vi "process.vi"(8 "error in":errorcluster, 9 "result allocation":T2, 10 "parameters":T2, 11 "Simple Sequencer TBM runtime in":refnum<class "Simple Sequencer TBM runtime.lvclass">) -> (0 "error out":errorcluster, 1 "results":T2, 2 "parameter allocation":T2, 3 "Simple Sequencer TBM runtime out":refnum<class "Simple Sequencer TBM runtime.lvclass">)   [LabVIEW 2015, in "Simple Sequencer TBM runtime.lvclass"]
doc: "Provides an interface for information processing by a module at runtime. While this interface performs no operations, a child should provide an override which may process data in any manner necessary."
uses:
  Simple Sequencer TBM runtime.lvclass
  <vilib>/NI/Tag Bus/table/data table.ctl
  sequencer states.ctl
  Simple Sequencer TBM runtime.lvclass/Simple Sequencer TBM runtime.ctl
  sequencer commands.ctl
  meta sequence definition.ctl
  <vilib>/NI/AMC/Read Termination Message.vi
  <vilib>/NI/AMC/Create Single Message.vi
  <vilib>/NI/AMC/Update Message Routing Info.vi
  <vilib>/NI/AMC/Globals.vi
  <vilib>/NI/AMC/Send Message.vi
  <vilib>/NI/AMC/AMC.lvlib
  <vilib>/NI/Tag Bus/table/data table.lvlib
panel:
  out "state":T1
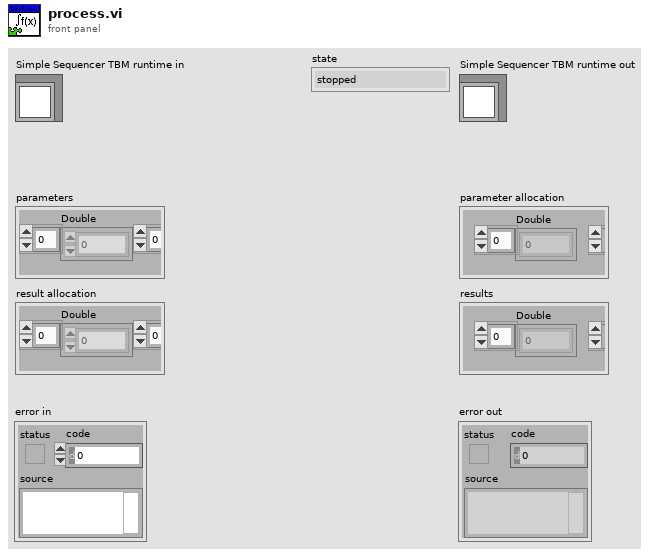
[diagram p1: front panel]
types:
  T1 = typedef "Simple Sequencer TBM runtime.lvclass/sequencer states.ctl" = enum16{"stopped", "running", "paused"}
  T2 = typedef "tag bus.lvlib/data table.lvlib/data table.ctl" = cluster{"Double":dbl[], "Single":sgl[], "I64":i64[], "I32":i32[], "I16":i16[], "I8":i8[], "U64":u64[], "U32":u32[], "U16":u16[], "U8":u8[], "Boolean":bool[], "String":string[], "Array of Double":cluster{"DBL Array":dbl[]}[], "Array of Single":cluster{"SGL Array":sgl[]}[], "Array of I64":cluster{"I64 Array":i64[]}[], "Array of I32":cluster{"I32 Array":i32[]}[], "Array of I16":cluster{"I16 Array":i16[]}[], "Array of I8":cluster{"I8 Array":i8[]}[], "Array of U64":cluster{"U64 Array":u64[]}[], "Array of U32":cluster{"U32 Array":u32[]}[], "Array of U16":cluster{"U16 Array":u16[]}[], "Array of U8":cluster{"U8 Array":u8[]}[], "Array of Boolean":cluster{"Boolean Array":bool[]}[], "Array of String":cluster{"String Array":string[]}[]}
  T3 = typedef "Simple Sequencer TBM runtime.lvclass/sequencer commands.ctl" = enum16{"Run", "Pause", "Resume", "Stop"}
  T4 = typedef "Simple Sequencer TBM runtime.lvclass/meta sequence definition.ctl" = cluster{"sequence length":i32, "sequence pointers":i32[], "continue location":i32}
  T5 = typedef "AMC.lvlib/Message Queue.ctl" = refnum<queue>
  T6 = typedef "Simple Sequencer TBM runtime.lvclass/sequence definition.ctl" = cluster{"sequence name":string, "sequence length":i32, "actions with configuration":T7[]}
  T7 = typedef "Simple Sequencer TBM runtime.lvclass/actions with configuration.ctl" = cluster{"action":refnum<class "action.lvclass">, "parameters":T2, "parameters specification":T8[], "results":T2, "results specification":T8[]}
  T8 = typedef "tag bus.lvlib/data table.lvlib/transfer specification.ctl" = cluster{"data type":T9, "sink indices":i32[], "source indices":i32[]}
  T9 = typedef "tag bus.lvlib/tag descriptor.lvclass/Data Type.ctl" = enum16{"Double", "Single", "I64", "I32", "I16", "I8", "U64", "U32", "U16", "U8", "Boolean", "String", "Array of Double", "Array of Single", "Array of I64", "Array of I32", "Array of I16", "Array of I8", "Array of U64", "Array of U32", "Array of U16", "Array of U8", "Array of Boolean", "Array of String"}
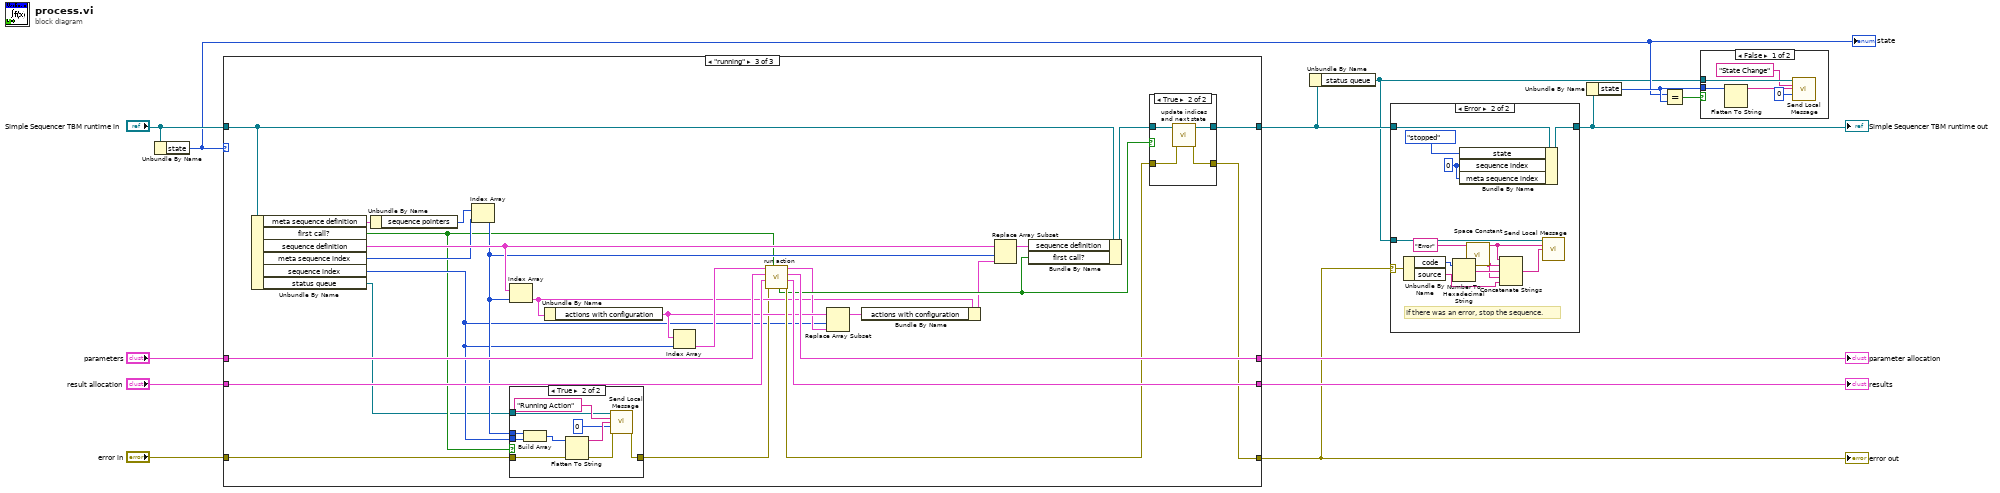
[diagram p0: block diagram]
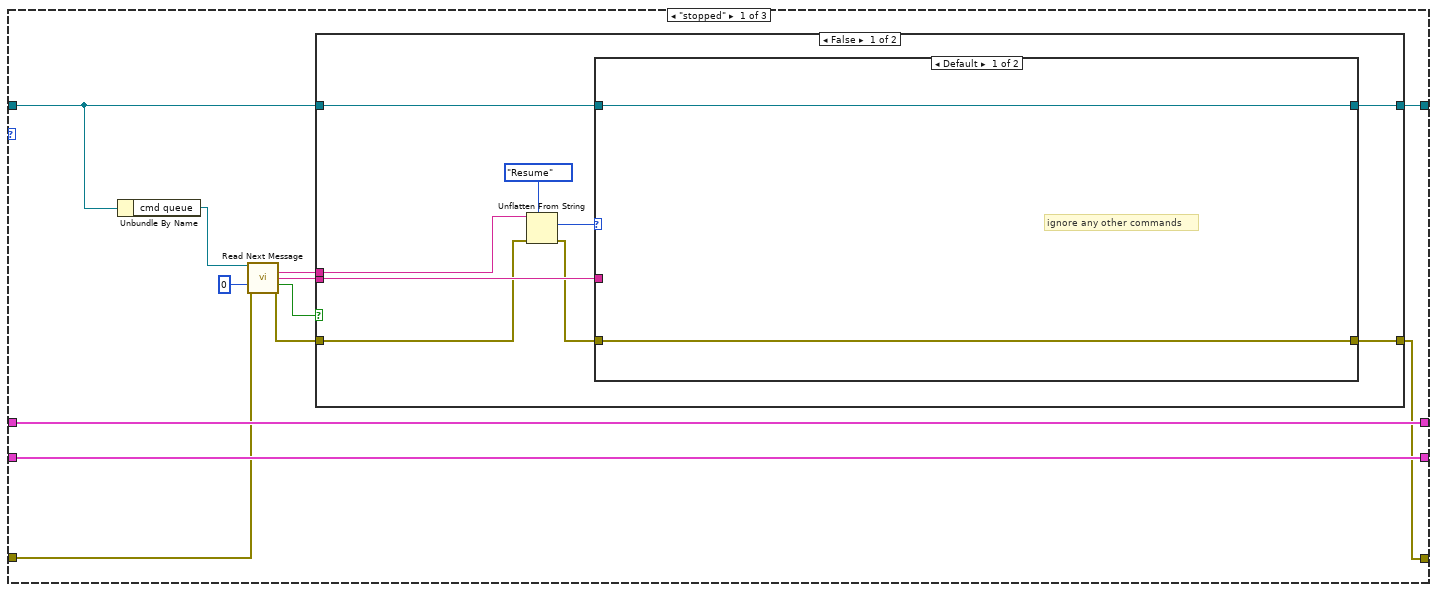
[diagram p4: hidden frame]
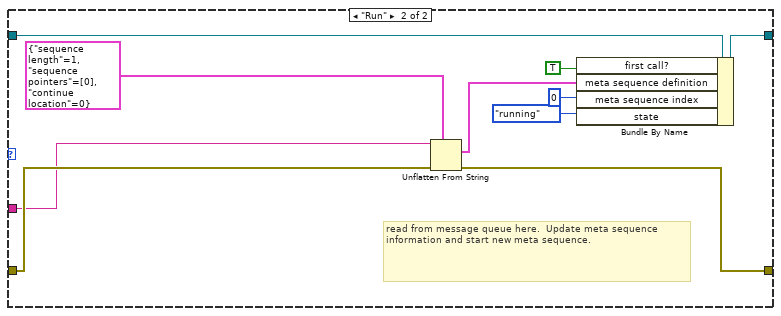
[diagram p5: hidden frame]
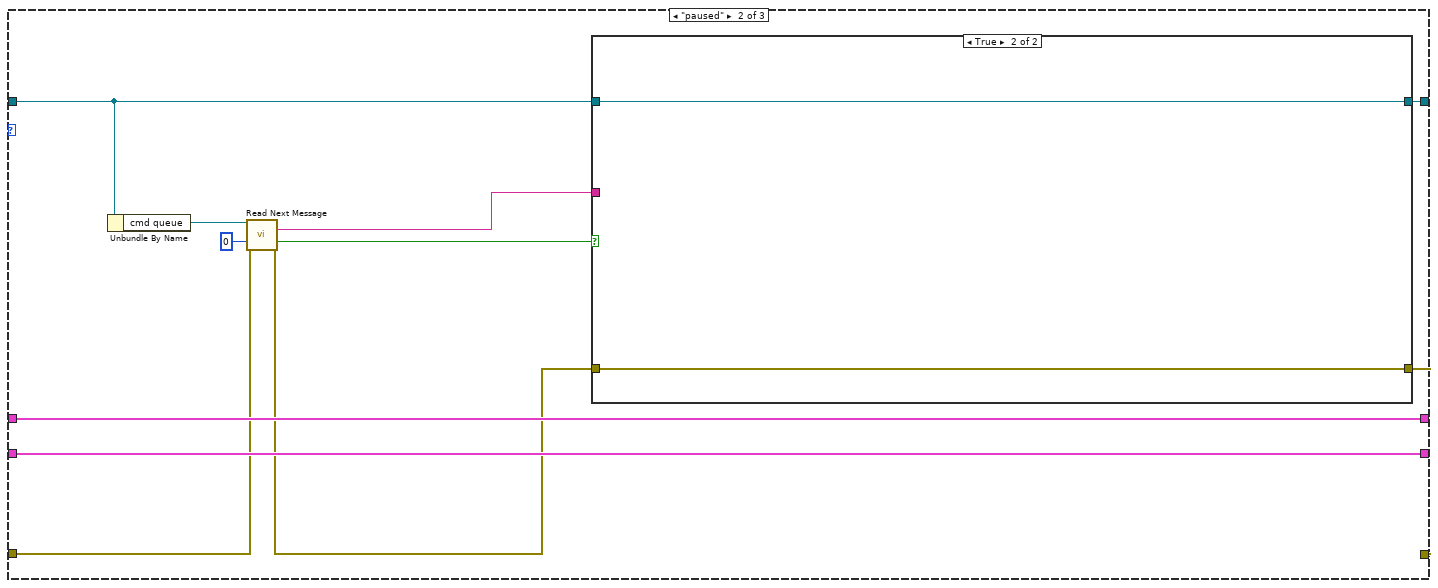
[diagram p7: hidden frame]
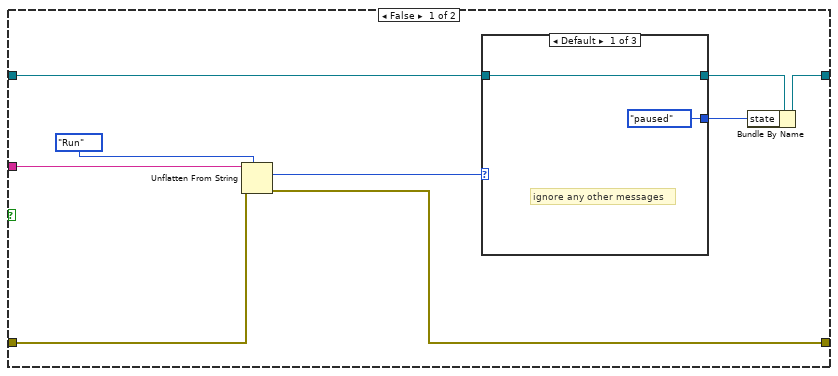
[diagram p8: hidden frame]
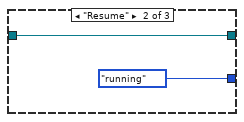
[diagram p9: hidden frame]
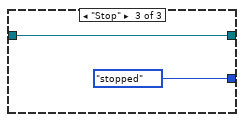
[diagram p10: hidden frame]
diagram:
  n1 = Unbundle By Name("Simple Sequencer TBM runtime in") -> ("state"=w5:T1)
  "state" <- w5
  n2 = case shown="\"running\"" w5 {
    tunnel: "Simple Sequencer TBM runtime in" -> [w22 w54 w83]
    tunnel: "error in" -> [w19 w55 w82]
    tunnel: [w16 w49 w94] -> w2
    tunnel: [w23 w53 w95] -> w4
    tunnel: "parameters" -> [w25 w59 w101]
    tunnel: "result allocation" -> [w24 w58 w100]
    tunnel: [w24 w58 w102] -> w10
    tunnel: [w25 w59 w103] -> w11
    frame "stopped" {
      n3 = Unbundle By Name(w22) -> ("cmd queue"=w21:T5)
      n4 = call <vilib>:"Read Next Message.vi"("message queue in"=w21, "timeout (1 ms)"=0, "error in"=w19) -> ("message name"=w14:string, "message value"=w17:string, "timed out?"=w18:bool, "error out"=w15:errorcluster)  [unwired: 5 in, 4 out]
      n5 = case shown="False" w18 {
        tunnel: [w34 w47] -> w23
        tunnel: w22 -> [w33 w47]
        tunnel: w17 -> [w32 _]
        tunnel: w15 -> [w28 w48]
        tunnel: [w31 w48] -> w16
        tunnel: w14 -> [w29 _]
        frame False {
          n6 = Unflatten From String(type=sequencer_commands."Resume" ("Commands"), binary string=w29, error in (no error)=w28) -> (value=w26:T3, error out=w27:errorcluster)  [unwired: 2 in, 1 out]
          n7 = case shown="Default" w26 {
            tunnel: [w35 w43] -> w34
            tunnel: w33 -> [w35 w42]
            tunnel: w32 -> [_ w37]
            tunnel: w27 -> [w36 w40]
            tunnel: [w36 w39] -> w31
            frame Default {
              # "ignore any other commands"
            }
            frame "Run" {
              # "read from message queue here.  Update meta sequence information and start new meta sequence."
              n8 = Unflatten From String(type=T4 {"sequence length"=1, "sequence pointers"=[0], "continue location"=0} ("meta sequence definition"), binary string=w37, error in (no error)=w40) -> (value=w38:T4, error out=w39:errorcluster)  [unwired: 2 in, 1 out]
              n9 = Bundle By Name(cluster=w42, "first call?"=TRUE, "meta sequence definition"=w38, "meta sequence index"=0, "state"=sequencer_states."running") -> (w43:refnum<class "Simple Sequencer TBM runtime.lvclass">)
            }
          }
        }
        frame True {
          # "stay stopped in the timeout case"
        }
      }
    }
    frame "paused" {
      n10 = Unbundle By Name(w54) -> ("cmd queue"=w56:T5)
      n11 = call <vilib>:"Read Next Message.vi"("message queue in"=w56, "timeout (1 ms)"=0, "error in"=w55) -> ("message name"=w51:string, "timed out?"=w52:bool, "error out"=w50:errorcluster)  [unwired: 5 in, 5 out]
      n12 = case shown="True" w52 {
        tunnel: w54 -> [w68 w76]
        tunnel: [w66 w76] -> w53
        tunnel: w51 -> [w63 _]
        tunnel: w50 -> [w62 w75]
        tunnel: [w61 w75] -> w49
        frame False {
          n13 = Unflatten From String(type=sequencer_commands."Run" ("Commands"), binary string=w63, error in (no error)=w62) -> (value=w60:T3, error out=w61:errorcluster)  [unwired: 2 in, 1 out]
          n14 = case shown="Default" w60 {
            tunnel: w68 -> [w70 w72 w74]
            tunnel: [w70 w72 w74] -> w67
            tunnel: [sequencer_states."paused" ("state") sequencer_states."running" ("state") sequencer_states."stopped" ("state")] -> w65
            frame Default {
              # "ignore any other messages"
            }
            frame "Resume" {
            }
            frame "Stop" {
            }
          }
          n15 = Bundle By Name(cluster=w67, "state"=w65) -> (w66:refnum<class "Simple Sequencer TBM runtime.lvclass">)
        }
        frame True {
        }
      }
    }
    frame "running" {
      n16 = Unbundle By Name(w83) -> ("meta sequence definition"=w86:T4, "first call?"=w78:bool, "sequence definition"=w98:T6[], "meta sequence index"=w84:i32, "sequence index"=w79:i32, "status queue"=w77:T5)
      n17 = Unbundle By Name(w86) -> ("sequence pointers"=w85:i32[])
      n18 = Index Array(array=w85, index=w84) -> (element=w80:i32)
      n19 = Index Array(array=w98, index=w80) -> (element=w89:T6)
      n20 = case shown="True" w78 {
        tunnel: w82 -> [w104 w109]
        tunnel: [w104 w108] -> w81
        tunnel: w80 -> [_ w107]
        tunnel: w79 -> [_ w106]
        tunnel: w77 -> [_ w105]
        frame False {
        }
        frame True {
          n21 = Build Array(w107, w106) -> (w110:i32[])
          n22 = Flatten To String(anything=w110, error in (no error)=w109) -> (data string=w113:string, error out=w114:errorcluster)  [unwired: 2 in, 1 out]
          n23 = call <vilib>:"Send Local Message.vi"("message queue in"=w105, "message name"="Running Action", "message value"=w113, "timeout (-1 ms)"=0, "error in"=w114) -> ("error out"=w108:errorcluster)  [unwired: 8 in, 2 out]
        }
      }
      n24 = Unbundle By Name(w89) -> ("actions with configuration"=w91:T7[])
      n25 = Index Array(array=w91, index=w79) -> (element=w92:T7)
      n26 = call "run action.vi"("first call?"=w78, "error in (no error)"=w81, "result allocation"=w100, "parameters"=w101, "action with configuration"=w92) -> ("error out"=w99:errorcluster, "results"=w102:T2, "parameters allocation"=w103:T2, "action with configuration out"=w90:T7, "complete?"=w93:bool)  [unwired: 2 in]
      n27 = Replace Array Subset(array=w91, new element=w90, index=w79) -> (w88:T7[])
      n28 = Bundle By Name(cluster=w89, "actions with configuration"=w88) -> (w87:T6)
      n29 = Replace Array Subset(array=w98, new element=w87, index=w80) -> (w97:T6[])
      n30 = Bundle By Name(cluster=w83, "sequence definition"=w97, "first call?"=w93) -> (w96:refnum<class "Simple Sequencer TBM runtime.lvclass">)
      n31 = case shown="True" w93 {
        tunnel: w96 -> [w115 w120]
        tunnel: [w115 w117] -> w95
        tunnel: w99 -> [w116 w119]
        tunnel: [w116 w118] -> w94
        frame False {
        }
        frame True {
          n32 = call "update indices and next state.vi"("error in"=w119, "Simple Sequencer TBM runtime in"=w120) -> ("error out"=w118:errorcluster, "Simple Sequencer TBM runtime out"=w117:refnum<class "Simple Sequencer TBM runtime.lvclass">)  [unwired: 8 in]
        }
      }
    }
  }
  "error out" <- w2
  "results" <- w10
  "parameter allocation" <- w11
  n33 = Unbundle By Name(w4) -> ("status queue"=w1:T5)
  n34 = case shown="Error" w2 {
    selector: w2 -> [_ w128]
    tunnel: w4 -> [w121 w133]
    tunnel: [w121 w130] -> w3
    tunnel: w1 -> [_ w129]
    frame No Error {
    }
    frame Error {
      w127 = "Error" ("message name")
      w132 = 0 ("sequence index")
      # "If there was an error, stop the sequence."
      n35 = Unbundle By Name(w128) -> ("code"=w126:i32, "source"=w122:string)
      n36 = Number To Hexadecimal String(2:w126) -> (0:w124:string)  [unwired: 1 in]
      n37 = Bundle By Name(cluster=w133, "state"=sequencer_states."stopped" ("t"), "sequence index"=w132, "meta sequence index"=w132) -> (w130:refnum<class "Simple Sequencer TBM runtime.lvclass">)
      n38 = call <vilib>:"Space Constant.vi"() -> ("String"=w123:string)
      n39 = Concatenate Strings(w127, w123, w124, w123, w122) -> (w125:string)
      n40 = call <vilib>:"Send Local Message.vi"("message queue in"=w129, "message name"=w127, "message value"=w125) -> ()  [unwired: 10 in, 3 out]
    }
  }
  "Simple Sequencer TBM runtime out" <- w3
  n41 = Unbundle By Name(w3) -> ("state"=w8:T1)
  n42 = Equal?(x=w5, y=w8) -> (x = y?=w9:bool)
  n43 = case shown="False" w9 {
    tunnel: w1 -> [w138 _]
    tunnel: w8 -> [w136 _]
    frame False {
      n44 = Flatten To String(anything=w136) -> (data string=w135:string)  [unwired: 3 in, 2 out]
      n45 = call <vilib>:"Send Local Message.vi"("message queue in"=w138, "message name"="State Change", "message value"=w135, "timeout (-1 ms)"=0) -> ()  [unwired: 9 in, 3 out]
    }
    frame True {
    }
  }
